vi "Read Unicode from String Control.vi"() -> ()   [LabVIEW 2009]
panel:
  in  "stop":bool
  in  "Display as Unicode":bool
  out "String":string="Hello World"
  in  "Input String (Force Unicode on)":string="H\u0000e\u0000l\u0000l\u0000o\u0000 \u0000W\u0000o\u0000r\u0000l\u0000d\u0000"
  out "ASCII":string
  out "Unicode":string
  out "byte stream (hex)":u8[](array[numeric])=[72, 0, 101, 0, 108, 0, 108, 0, 111, 0, 32, 0, 87, 0, 111, 0, 114, 0, 108, 0, 100, 0] format="%.0x"
  out "Hex":string
  out "Hex":string="Hello World"
  out "byte stream (hex)":u8[](array[numeric])=[72, 101, 108, 108, 111, 32, 87, 111, 114, 108, 100] format="%.0x"
  out "Unicode":string="Hello World"
  out "ASCII":string="Hello World"
  in  "Input String (Force Unicode off)":string="Hello World"
  # "This control is set to Unicode display mode programmatically after every value change (key stroke). The 'Update Value while Typing' property is turned on."
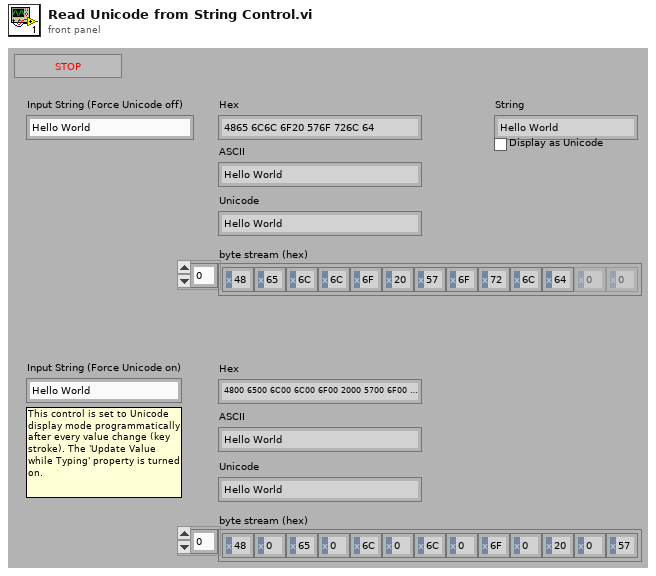
[diagram p1: front panel]
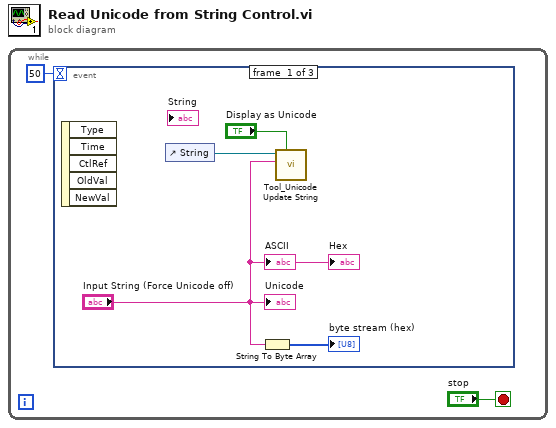
[diagram p0: block diagram]
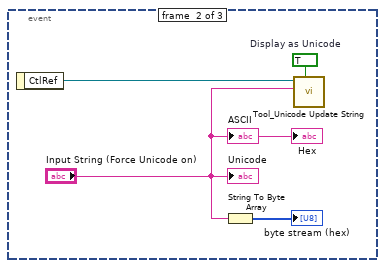
[diagram p2: hidden frame]
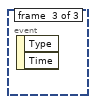
[diagram p3: hidden frame]
diagram:
  n1 = while {
    stop <- "stop" stop-if-true
    n2 = event shown="[1] \"Input String (Force Unicode on)\": Value Change" {
      selector: _ -> [_ _ _]
      dyn-events: _ -> [_ _ _]
      timeout: 50 -> [_ _ _]
      event #0 {
        n3 = event-data() -> ()  [unwired: 1 in, 5 out]
        n4 = control-ref of="String"() -> (w4:refnum<vi>)
        n5 = String To Byte Array(string="Input String (Force Unicode off)") -> (unsigned byte array=→"byte stream (hex)":u8[])
        n6 = call "Tool_Unicode Update String.vi"("Interpret as Unicode (T)"="Display as Unicode", "String Value"="Input String (Force Unicode off)", "String Control Reference"=w4) -> ()  [unwired: 5 in, 2 out]
        "ASCII" <- "Input String (Force Unicode off)"
        "Unicode" <- "Input String (Force Unicode off)"
        "Hex" <- "Input String (Force Unicode off)"
      }
      event #1 {
        w9 = TRUE  # Display as Unicode
        n7 = event-data() -> ("CtlRef"=w8:refnum<vi>)  [unwired: 1 in]
        n8 = String To Byte Array(string="Input String (Force Unicode on)") -> (unsigned byte array=→"byte stream (hex)":u8[])
        n9 = call "Tool_Unicode Update String.vi"("Interpret as Unicode (T)"=w9, "String Value"="Input String (Force Unicode on)", "String Control Reference"=w8) -> ()  [unwired: 5 in, 2 out]
        "ASCII" <- "Input String (Force Unicode on)"
        "Unicode" <- "Input String (Force Unicode on)"
        "Hex" <- "Input String (Force Unicode on)"
      }
      event #2 {
        n10 = event-data() -> ()  [unwired: 1 in, 2 out]
      }
    }
  }
